vi "CNR.vi"(0 "Image In":T2, 1 "Background Size (25)":i32=41, 5 "Point":T1 {"Y" format="%.2f"; "X" format="%.2f"}, 7 "Search Area (11)":i32=11, 9 "Hole ROI Size (3)":i32=5, 12 "Cut (11)":i32=21) -> (2 "Hole":T2, 3 "CNR Point":T1 {"Y" format="%.2f"; "X" format="%.2f"}, 4 "CNR":dbl=2.6081367311632224, 6 "Max SNR":dbl, 8 "Median in Hole":dbl, 10 "Mean Backround":dbl, 13 "Background":T2, 14 "Image":T2(plugin-control), 15 "StdDev in Background":dbl)   [LabVIEW 2023]
uses:
  <vilib>/vision/Image Controls.llb/IMAQ Image.ctl
  <vilib>/vision/NI_Vision_Development_Module.lvlib
  <vilib>/Analysis/NI_AALBase.lvlib
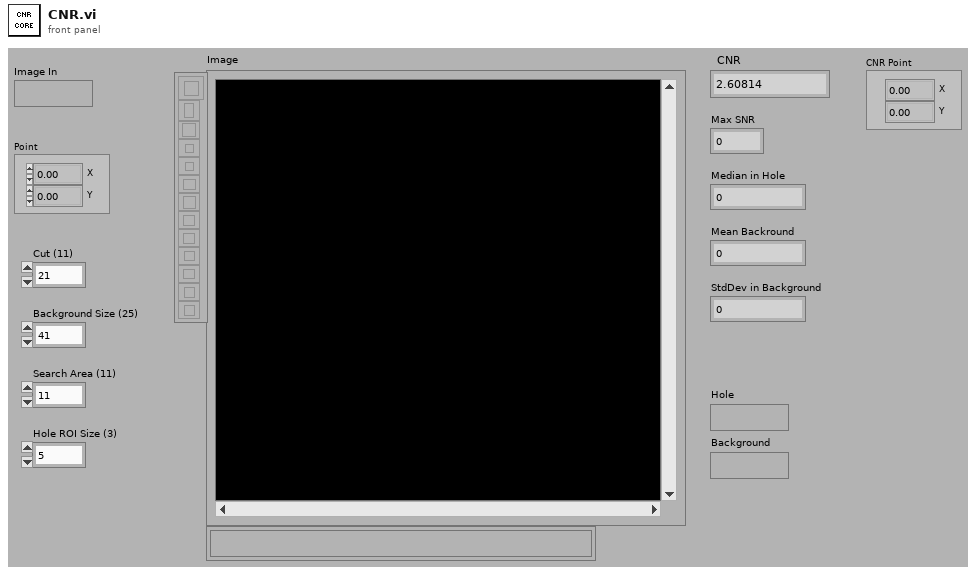
[diagram p1: front panel]
types:
  T1 = typedef "IMAQ Point" = cluster{"X":sgl, "Y":sgl}
  T2 = typedef "IMAQ Image.ctl" = refnum<image>
  T3 = typedef "Image Type" = u32
  T4 = cluster{"[0]":i32, "[1]":i32, "[2]":i32, "[3]":i32}
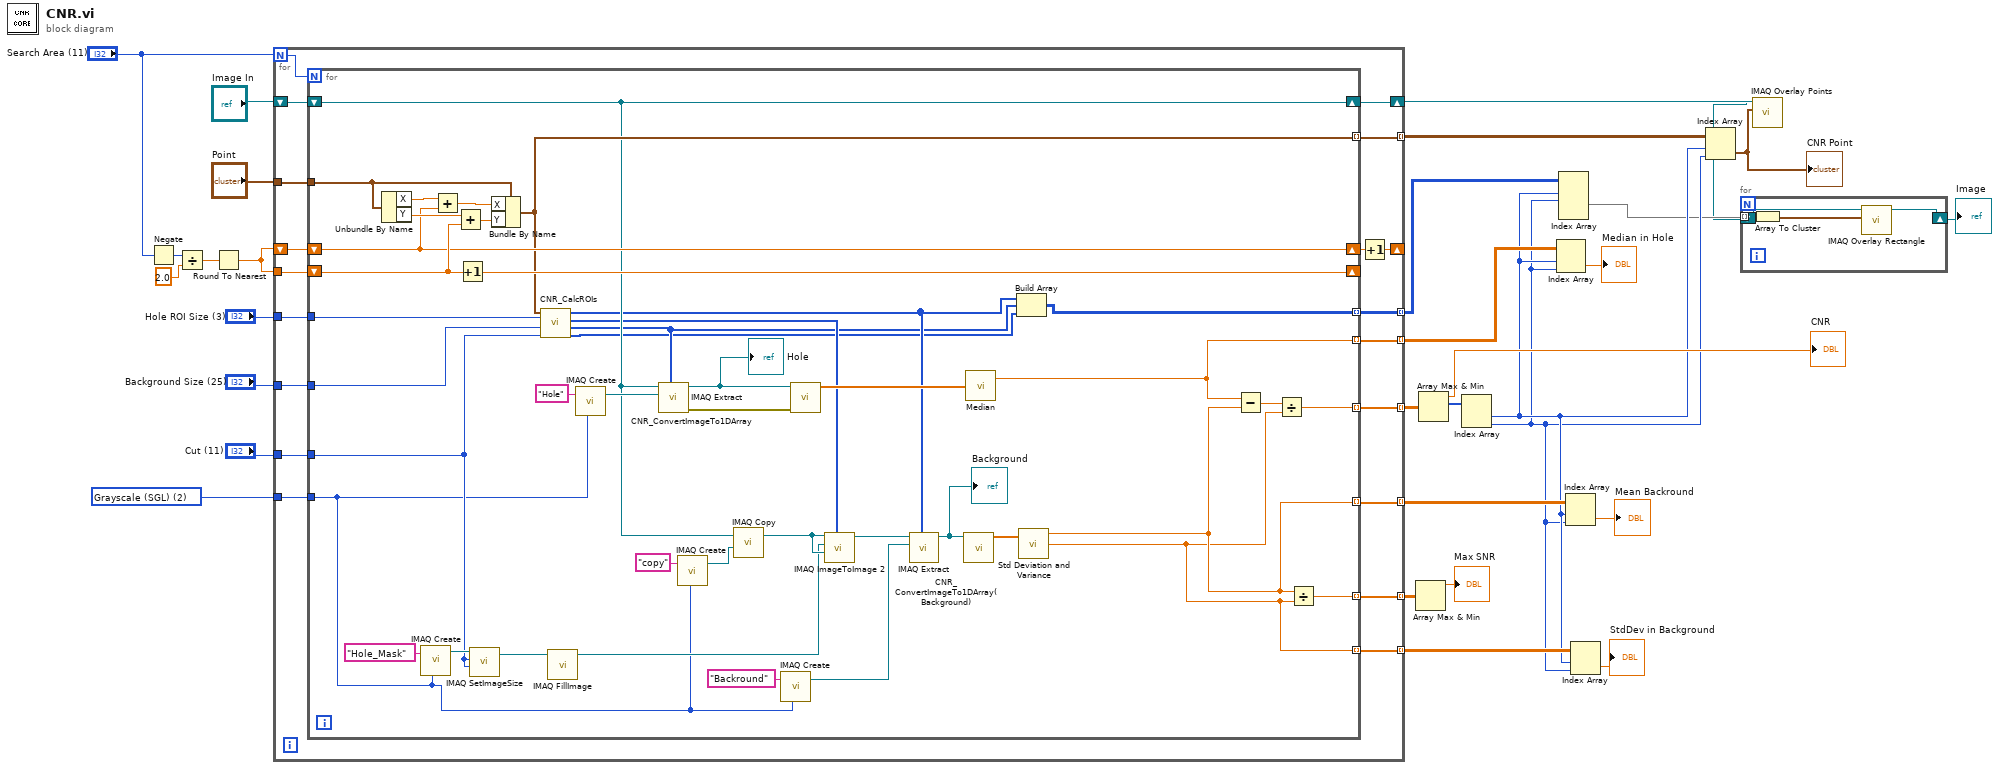
[diagram p0: block diagram]
diagram:
  w7 = T3 2 items=["Grayscale (U8)", "Grayscale (I16)", "Grayscale (SGL)", "Complex (CSG)", "RGB (U32)", "HSL (U32)", "RGB (U64)", "Grayscale (U16)"] ("Image Type")
  n1 = Negate(x="Search Area (11)") -> (-x=w26:i32)
  n2 = Divide(x=w26, y=sgl 2.0) -> (x/y=w25:sgl)
  n3 = Round To Nearest(number=w25) -> (nearest integer value=w18:sgl)
  n4 = for {
    N: "Search Area (11)" -> [w49]
    tunnel: "Point" -> [w50]
    shift-right: [w44] -> _
    shift-left: w18 -> [w48]
    tunnel: w18 -> [w47]
    tunnel: [w46] -> w23 mode=indexing
    tunnel: [w43] -> w30 mode=indexing
    tunnel: [w41] -> w22 mode=indexing
    shift-right: [w40] -> w17
    shift-left: "Image In" -> [w42]
    tunnel: "Hole ROI Size (3)" -> [w39]
    tunnel: "Background Size (25)" -> [w38]
    tunnel: "Cut (11)" -> [w37]
    tunnel: [w36] -> w8 mode=indexing
    tunnel: [w35] -> w13 mode=indexing
    tunnel: [w34] -> w11 mode=indexing
    tunnel: w7 -> [w33]
    tunnel: [w32] -> w6 mode=indexing
    n5 = for {
      N: w49 -> [_]
      tunnel: w50 -> [w77]
      shift-right: [w69] -> w45
      shift-left: w48 -> [w69]
      shift-right: [w75] -> _
      shift-left: w47 -> [w73]
      tunnel: [w70] -> w46 mode=indexing
      tunnel: [w68] -> w43 mode=indexing
      tunnel: [w66] -> w41 mode=indexing
      shift-right: [w64] -> w40
      shift-left: w42 -> [w64]
      tunnel: w39 -> [w63]
      tunnel: w38 -> [w62]
      tunnel: w37 -> [w61]
      tunnel: [w60] -> w36 mode=indexing
      tunnel: [w59] -> w35 mode=indexing
      tunnel: [w58] -> w34 mode=indexing
      tunnel: w33 -> [w56]
      tunnel: [w51] -> w32 mode=indexing
      n6 = Unbundle By Name(w77) -> ("X"=w76:sgl, "Y"=w74:sgl)
      n7 = call "IMAQ Create"("Image Name"="Hole_Mask", "Image Type"=w56) -> ("New Image"=w84:T2)  [unwired: 3 in, 1 out]
      n8 = Add(x=w76, y=w69) -> (x+y=w72:sgl)
      n9 = Add(x=w74, y=w73) -> (x+y=w71:sgl)
      n10 = Increment(x=w73) -> (x+1=w75:sgl)
      n11 = call "IMAQ SetImageSize"("Y Resolution"=w61, "X Resolution"=w61, "Image"=w84) -> ("Image Out"=w83:T2)  [unwired: 2 in, 1 out]
      n12 = Bundle By Name(cluster=w77, "X"=w72, "Y"=w71) -> (w68:T1)
      n13 = call "CNR_CalcROIs.vi"("Cut"=w61, "Background Size"=w62, "LOCH ROI Size"=w63, "Point"=w68) -> ("CutOff ROI"=w52:i32[], "Hole ROI"=w53:i32[], "Mask Insertion Point"=w55:i32[], "Background ROI"=w54:i32[])  [unwired: 4 in]
      n14 = call "IMAQ FillImage"("Image"=w83) -> ("Image Out"=w82:T2)  [unwired: 9 in, 1 out]
      n15 = call "IMAQ Create"("Image Name"="Hole", "Image Type"=w56) -> ("New Image"=w91:T2)  [unwired: 3 in, 1 out]
      n16 = call "IMAQ Extract"("Optional Rectangle"=w53, "Image Dst"=w91, "Image Src"=w64) -> ("error out"=w65:errorcluster, "Image Dst Out"=w67:T2)  [unwired: 7 in]
      "Hole" <- w67
      n17 = call "IMAQ Create"("Image Name"="copy", "Image Type"=w56) -> ("New Image"=w87:T2)  [unwired: 3 in, 1 out]
      n18 = call "IMAQ Copy"("Image Dst"=w87, "Image Src"=w64) -> ("Image Dst Out"=w86:T2)  [unwired: 4 in, 1 out]
      n19 = call "IMAQ Create"("Image Name"="Backround", "Image Type"=w56) -> ("New Image"=w89:T2)  [unwired: 3 in, 1 out]
      n20 = call "CNR_ConvertImageTo1DArray.vi"("error in (no error)"=w65, "Refnum in"=w67) -> ("Array"=w78:dbl[])  [unwired: 8 in, 1 out]
      n21 = call "IMAQ ImageToImage 2"("Offset Left/Top"=w55, "Image Dst"=w86, "Image Src (Small)"=w82, "Image Src (Large)"=w86) -> ("Image Dst Out"=w81:T2)  [unwired: 6 in, 1 out]
      n22 = call "IMAQ Extract"("Optional Rectangle"=w54, "Image Dst"=w89, "Image Src"=w81) -> ("Image Dst Out"=w79:T2)  [unwired: 7 in, 1 out]
      "Background" <- w79
      n23 = call "CNR_ConvertImageTo1DArray(Background).vi"("Refnum in"=w79) -> ("Array"=w57:dbl[])  [unwired: 9 in, 1 out]
      n24 = call <vilib>:"Median.vi"("X"=w78) -> ("median"=w60:dbl)  [unwired: 1 out]
      n25 = Build Array(w54, w53, w52) -> (w51:i32[][])
      n26 = call <vilib>:"Std Deviation and Variance.vi"("X"=w57) -> ("mean"=w59:dbl, "standard deviation"=w58:dbl)  [unwired: 1 in, 1 out]
      n27 = Subtract(x=w60, y=w59) -> (x-y=w80:dbl)
      n28 = Divide(x=w80, y=w58) -> (x/y=w70:dbl)
      n29 = Divide(x=w59, y=w58) -> (x/y=w66:dbl)
    }
    n30 = Increment(x=w45) -> (x+1=w44:sgl)
  }
  n31 = Array Max & Min(array=w22) -> (max value=→"Max SNR":dbl)  [unwired: 3 out]
  n32 = Array Max & Min(array=w23) -> (max value=→"CNR":dbl, max index (indices)=w29:i32[])  [unwired: 2 out]
  n33 = Index Array(array=w29) -> (element #1=w5:i32, element #2=w4:i32)  [unwired: 2 in]
  n34 = Index Array(array=w8, index (row)=w5, index (col)=w4) -> (element=→"Median in Hole":dbl)
  n35 = Index Array(array=w6, index (dim 0)=w5, index (dim 1)=w4) -> (element=w3:i32[][])  [unwired: 2 in]
  n36 = Index Array(array=w13, index (row)=w5, index (col)=w4) -> (element=→"Mean Backround":dbl)
  n37 = Index Array(array=w11, index (row)=w5, index (col)=w4) -> (element=→"StdDev in Background":dbl)
  n38 = Index Array(array=w30, index (row)=w5, index (col)=w4) -> (element=w28:T1)
  "CNR Point" <- w28
  n39 = call "IMAQ Overlay Points"("Point"=w28, "Image"=w17) -> ("Image Out"=w2:T2)  [unwired: 8 in, 1 out]
  n40 = for {
    tunnel: w3 -> [w96] mode=indexing
    shift-right: [w93] -> w1
    shift-left: w2 -> [w94]
    n41 = Array To Cluster(array=w96) -> (cluster=w95:T4)
    n42 = call "IMAQ Overlay Rectangle"("Rectangle"=w95, "Image"=w94) -> ("Image Out"=w93:T2)  [unwired: 8 in, 1 out]
  }
  "Image" <- w1
